vi "Global_var.vi"() -> ()   [LabVIEW 2019]
panel:
  in  "com_erp42":refnum<visa-resource-name>="COM4"
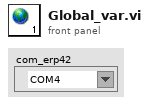
[diagram p1: front panel]
diagram:
